vi "UART.vi"(10 "DIO Refnum":refnum<k21>, 11 "Refnum in":refnum<k21>) -> ()   [LabVIEW 2019]
uses:
  <vilib>/rvi/DataTransferAndStorage/Container/Common/niFpgaContainerExecOnDevCompGetState.vi
  <vilib>/rvi/Emulation/niFpgaEmulationIsFPGAContextNoSignature.vi
  <vilib>/rvi/Emulation/niFpgaSctlEmulationGetInTimedLoop.vi
  <vilib>/rvi/errors/niFpgaSetErrorForExecOnDevCompSimple.vi
  <vilib>/rvi/eio/common/nirviEmuReportErrorAndStop.vi
  <vilib>/rvi/DataTransferAndStorage/Container/Common/niFpgaContainerGetUniqueNameForEmu.vi
  <vilib>/rvi/FIFO/Fifo_Resource/nirvififoEmulationSetSize.vi
  <vilib>/rvi/FIFO/Fifo_Resource/nirviFifoEmulationQueueMgr.vi
  <instcachedir>/0/nirviFifoEmulationQueueMgr_E5CAEC123FF24DC58D834DCA3CDAA9B5.lvgen/nirviFifoEmulationQueueMgr_E5CAEC123FF24DC58D834DCA3CDAA9B5_001.vi
  <vilib>/rvi/FIFO/Fifo_Resource/nirvififoEmulationDetermineInputValidOut.vi
  <vilib>/rvi/FIFO/Fifo_Resource/nirvififoEmulationCreateLock.vi
  <vilib>/rvi/Emulation/niFpgaProcessEmulError.vi
  <vilib>/rvi/FIFO/Fifo_Resource/nirvififoEmulationObtainLock.vi
  <vilib>/rvi/FIFO/Fifo_Resource/nirvififoEmulationReleaseLock.vi
  <vilib>/rvi/occurrence/nirviWaitOnOccurrenceBase.vi
  <vilib>/rvi/errors/nirviReportUnexpectedCaseInternalError.vi
  <vilib>/rvi/errors/nirviReportUnexpectedCaseInternalError (U32).vi
  <vilib>/Utility/error.llb/Clear Errors.vi
  <vilib>/rvi/interface/RandomDataEmulation/niFpgaRandomDataHandleErrors.vi
  <vilib>/rvi/DataTransferAndStorage/Container/XNode/niFpgaContainer.xnode
  <vilib>/rvi/FIFO/Fifo_Resource/niFpgaFifoEmulationRefIn.vi
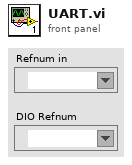
[diagram p1: front panel]
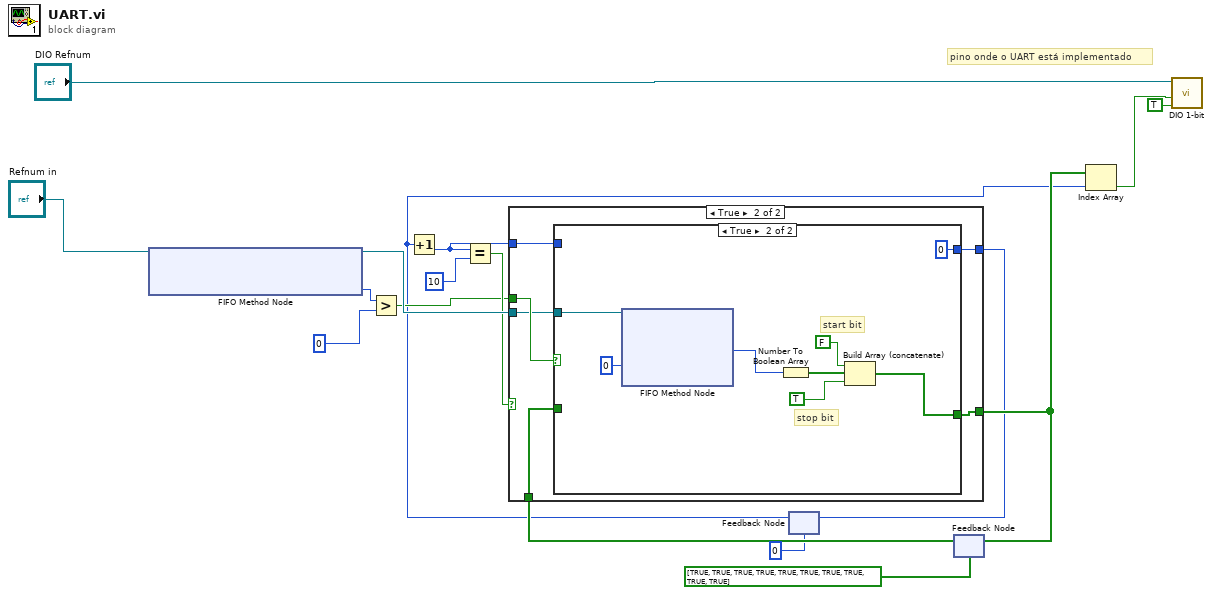
[diagram p0: block diagram]
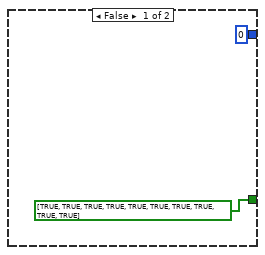
[diagram p3: hidden frame]
diagram:
  # "pino onde o UART está implementado"
  n1 = xnode ("FIFO Method Node")("FIFO In"="Refnum in") -> ("Number of Elements to Read"=w10:u32, "FIFO Out"=w17:refnum<k21>)
  n2 = Greater?(x=w10, y=u32 0) -> (0:w11:bool)
  n3 = feedback #1(u8 0) -> (w7:u8)
  n4 = Increment(x=w7) -> (x+1=w6:u8)
  n5 = Equal?(x=w6, y=u8 10) -> (x = y?=w15:bool)
  n6 = feedback #2(bool[] [TRUE, TRUE, TRUE, TRUE, TRUE, TRUE, TRUE, TRUE, TRUE, TRUE]) -> (w13:bool[])
  n7 = case shown="True" w15 {
    tunnel: [w18 w25] -> w5
    tunnel: w6 -> [w18 w24]
    tunnel: w11 -> [_ w21]
    tunnel: [w19 w23] -> w12
    tunnel: w13 -> [w19 w22]
    tunnel: w17 -> [_ w20]
    frame False {
    }
    frame True {
      n8 = case shown="True" w21 {
        tunnel: [u8 0 u8 0] -> w25
        tunnel: w24 -> [_ _]
        tunnel: [bool[] [TRUE, TRUE, TRUE, TRUE, TRUE, TRUE, TRUE, TRUE, TRUE, TRUE] w30] -> w23
        tunnel: w22 -> [_ _]
        tunnel: w20 -> [_ w28]
        frame False {
        }
        frame True {
          # "stop bit"
          # "start bit"
          n9 = xnode ("FIFO Method Node")("Timeout"=0, "FIFO In"=w28) -> ("Element"=w31:u8)  [unwired: 2 out]
          n10 = Number To Boolean Array(number=w31) -> (Boolean array=w33:bool[])
          n11 = Build Array (concatenate)(FALSE, w33, TRUE ("element")) -> (w30:bool[])
        }
      }
    }
  }
  n12 = feedback-in #1(w5) -> ()
  n13 = feedback-in #2(w12) -> ()
  n14 = Index Array(array=w12, index=w7) -> (element=w8:bool)
  n15 = call "DIO 1-bit.vi"("DIR"=TRUE, "OUT"=w8, "DIO Refnum"="DIO Refnum") -> ()  [unwired: 8 in, 1 out]
